vi "LOx_Pressure.vi"() -> ()   [LabVIEW 2018]
panel:
  out "Waveform Chart":dynamicdata(graph)
  out "?":dbl
  out "LOx Pressure":dbl(knob) scale=0.0..1500.0
  in  "End Loop":bool
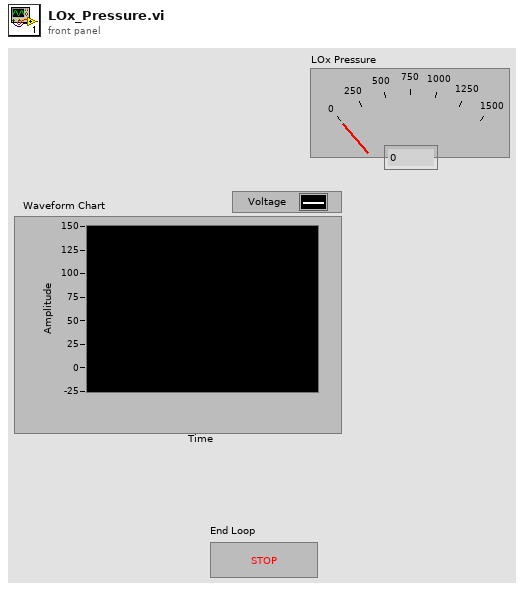
[diagram p1: front panel]
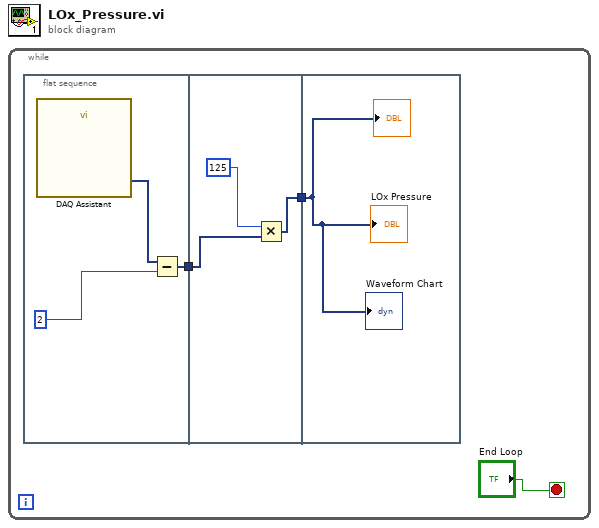
[diagram p0: block diagram]
diagram:
  n1 = while {
    stop <- "End Loop" stop-if-true
    n2 = flat-sequence {
      tunnel: [w5] -> w3
      tunnel: w3 -> [w8]
      tunnel: [w9] -> w2
      tunnel: w2 -> [w10]
      frame #0 {
        n3 = call "DAQ Assistant"() -> ("data"=w4:dynamicdata)  [unwired: 17 in, 2 out]
        n4 = Subtract(x=w4, y=2) -> (x-y=w5:dynamicdata)
      }
      frame #1 {
        n5 = Multiply(x=125, y=w8) -> (x*y=w9:dynamicdata)
      }
      frame #2 {
        "LOx Pressure" <- w10
        "?" <- w10
        "Waveform Chart" <- w10
      }
    }
  }
